vi "ToRepo.vi"(8 "error in":errorcluster, 9 "to repo cluster":T1, 10 "repository in":refnum<class "NISE_CEF_Repository.lvclass">, 11 "Systems in":refnum<class "Systems.lvclass">) -> (0 "error out":errorcluster, 2 "repository out":refnum<class "NISE_CEF_Repository.lvclass">, 3 "Systems out":refnum<class "Systems.lvclass">)   [LabVIEW 2013, in "PL Framework Configuration Tool.lvlib" / "Systems.lvclass"]
doc: "Transfers the information from the tree node into the repo. How it is stored in the repo depends on the Repo."
uses:
  Systems.lvclass
  <vilib>/CEF_TreeControl/Repository/NISE_CEF_Repository.lvclass
  <vilib>/CEF_TreeControl/Node/ToRepoCluster.ctl
  SystemConfigRepo/SystemConfigRepo.lvclass
  Framework Configuration Classes/platypus configuration/targets cluster.ctl
  Framework Configuration Classes/target configuration/PL_Target Configuration.lvclass
  Framework Configuration Classes/platypus configuration/engines cluster.ctl
  <vilib>/NI/Module Execution Interface/Engine Configuration/engine configuration.lvclass
  <vilib>/NI/Tag Bus Module Framework/module configuration/TBM module configuration.lvclass
  TBM Configuration Node/TBM Configuration Node.lvclass
  Systems.lvclass/Systems.ctl
  Framework Configuration Classes/system configuration/PL_System Configuration.lvclass/PL_System Configuration.ctl
  SystemConfigRepo/SystemConfigRepo.lvclass/SystemConfigRepo.ctl
  Framework Configuration Classes/system configuration/Write save time.vi
  <vilib>/NI/Tag Bus Module Framework/root configuration/set metadata property.vi
  Framework Configuration Classes/platypus configuration/PLConfigurationSerializer.lvlib
  Framework Configuration Classes/system configuration/PL_System Configuration.lvclass
  <vilib>/CEF_TreeControl/Node/NISE_CEF_Node.lvclass
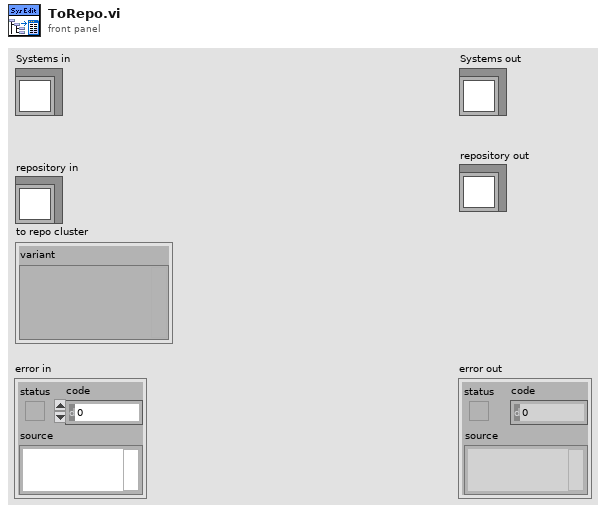
[diagram p1: front panel]
types:
  T1 = typedef "NISE_CEF_Node.lvclass/ToRepoCluster.ctl" = cluster{"variant":variant}
  T2 = typedef "PLConfigurationSerializer.lvlib/targets cluster.ctl" = cluster{"Target Configuration":refnum<class "PL_Target Configuration.lvclass">, "engines":T3[]}
  T3 = typedef "PLConfigurationSerializer.lvlib/engines cluster.ctl" = cluster{"engine configuration":refnum<class "engine configuration.lvclass">, "modules":refnum<class "TBM module configuration.lvclass">[]}
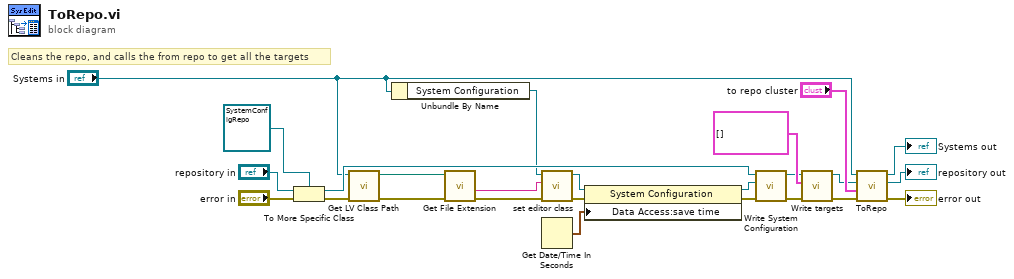
[diagram p0: block diagram]
diagram:
  # "Cleans the repo, and calls the from repo to get all the targets"
  n1 = To More Specific Class(target class=refnum<class "SystemConfigRepo.lvclass"> refnum ("SystemConfigRepo.lvclass"), reference="repository in", error in="error in") -> (specific class reference=w13:refnum<class "SystemConfigRepo.lvclass">, error out=w9:errorcluster)
  n2 = call <vilib>:"Get LV Class Path.vi"("error in (no error)"=w9, "object"="Systems in") -> ("error out"=w12:errorcluster, "class path"=w11:path)  [unwired: 8 in]
  n3 = Unbundle By Name("Systems in") -> ("System Configuration"=w8:refnum<class "PL_System Configuration.lvclass">)
  n4 = call <vilib>:"Get File Extension.vi"("error in (no error)"=w12, "file"=w11) -> ("error out"=w7:errorcluster, "filename without extension"=w5:string)  [unwired: 6 in, 2 out]
  n5 = call "set editor class.vi"("error in"=w7, "editor class"=w5, "configuration in"=w8) -> ("error out"=w6:errorcluster, "configuration out"=w3:refnum<class "PL_System Configuration.lvclass">)  [unwired: 7 in]
  n6 = Get Date/Time In Seconds() -> (seconds since 1Jan1904=w1:timestamp)
  n7 = property class="System Configuration"(reference=w3, error in=w6, "Data Access:save time"=w1) -> (reference out=w2:refnum<class "PL_System Configuration.lvclass">, error out=w4:errorcluster)
  n8 = call "Write System Configuration.vi"("error in"=w4, "System Configuration"=w2, "SystemConfigRepo in"=w13) -> ("error out"=w17:errorcluster, "SystemConfigRepo out"=w16:refnum<class "SystemConfigRepo.lvclass">)  [unwired: 7 in]
  n9 = call "Write targets.vi"("error in"=w17, "targets"=T2[] [], "SystemConfigRepo in"=w16) -> ("error out"=w14:errorcluster, "SystemConfigRepo out"=w15:refnum<class "SystemConfigRepo.lvclass">)  [unwired: 7 in]
  n10 = call-parent "ToRepo.vi"("error in"=w14, "to repo cluster"="to repo cluster", "repository in"=w15, "node in"="Systems in") -> ("error out"=→"error out":errorcluster, "repository out"=→"repository out":refnum<class "NISE_CEF_Repository.lvclass">, "node out"=→"Systems out":refnum<class "Systems.lvclass">)  [unwired: 5 in]
